vi "turn_rate_angle_test.vi"() -> ()   [LabVIEW 2009]
panel:
  out "Waveform Chart 2":dbl(graph)
  out "difference":dbl
  out "s? t:f":dbl
  out "Waveform Chart":dbl(graph)
  in  "Reverse":bool=TRUE
  in  "stop":bool
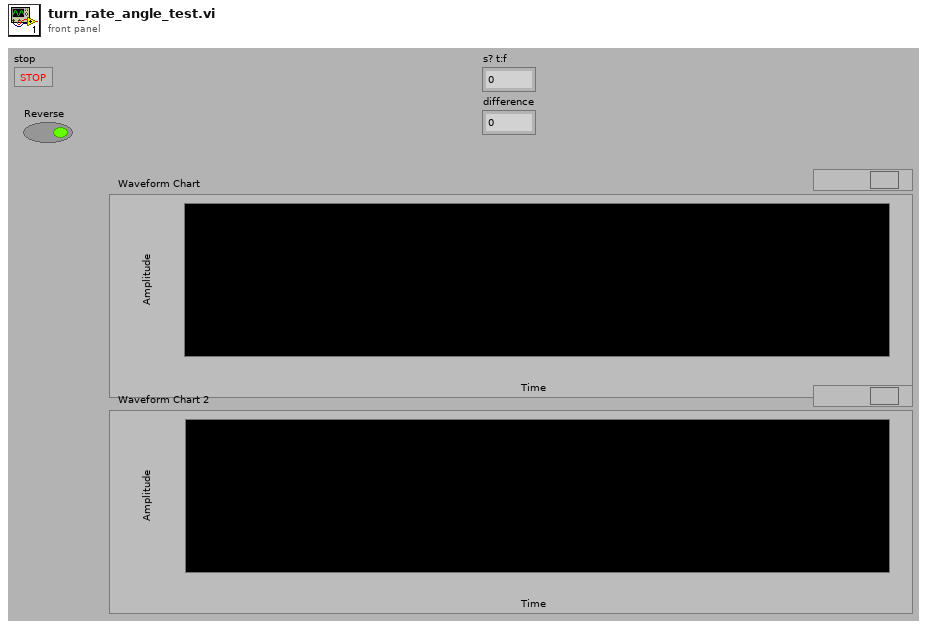
[diagram p1: front panel]
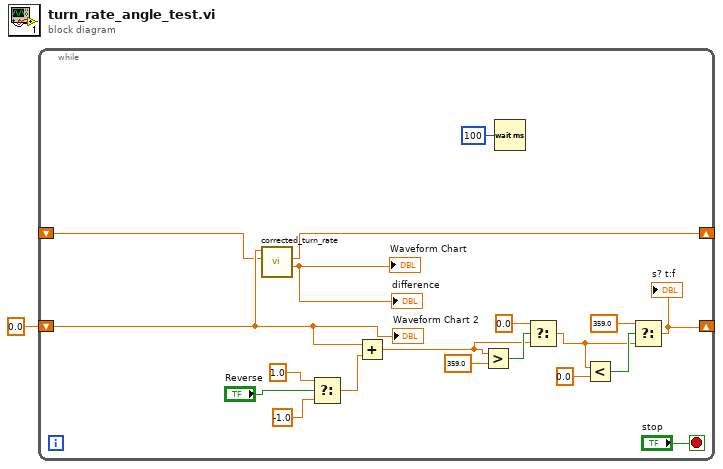
[diagram p0: block diagram]
diagram:
  n1 = while {
    shift-right: [w11] -> _
    shift-left: 0.0 -> [w4]
    shift-right: [w3] -> _
    shift-left: _ -> [w2]
    stop <- "stop" stop-if-true
    n2 = call "corrected_turn_rate.vi"("Previous Heading"=w2, "Current Heading"=w4) -> ("difference"=→"Waveform Chart" →"difference":dbl, "Current Heading"=w3:dbl)  [unwired: 7 in, 1 out]
    n3 = Select(t=1.0, s="Reverse", f=-1.0) -> (s? t:f=w18:dbl)
    n4 = Add(x=w4, y=w18) -> (x+y=w8:dbl)
    n5 = Greater?(x=w8, y=359.0) -> (0:w10:bool)
    n6 = Wait (ms)(milliseconds to wait=u32 100) -> ()  [unwired: 1 out]
    n7 = Select(t=0.0, s=w10, f=w8) -> (s? t:f=w6:dbl)
    n8 = Less?(x=w6, y=0.0) -> (x < y?=w12:bool)
    n9 = Select(t=359.0, s=w12, f=w6) -> (s? t:f=w11:dbl)
    "s? t:f" <- w11
    "Waveform Chart 2" <- w4
  }
